vi "FileSend.vi"(8 "error in (no error)":errorcluster, 10 "(Empty=No Action)":path caption="File Name & Path", 11 "controller in":refnum<k24>) -> (0 "error out":errorcluster, 3 "controller out":refnum<k24>)   [LabVIEW 2010]
uses:
  c:/aerotech/controller/5.xx.xxx/ensemble/pc/labview/2010/bin/Aerotech.Ensemble.dll
  bin/Aerotech.Ensemble.dll
  c:/aerotech/controller/5.xx.xxx/ensemble/pc/labview/2010/bin/Aerotech.Ensemble.LabVIEW.dll
  bin/Aerotech.Ensemble.LabVIEW.dll
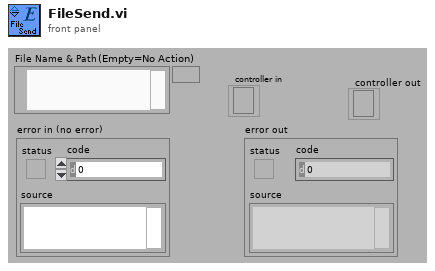
[diagram p1: front panel]
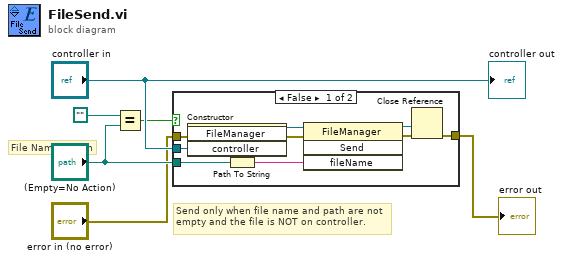
[diagram p0: block diagram]
diagram:
  # "File Name & Path"
  # "Send only when file name and path are not empty and the file is NOT on controller."
  n1 = Equal?(x=path "", y="(Empty=No Action)") -> (x = y?=w1:bool)
  n2 = case shown="False" w1 {
    tunnel: [w13 w16] -> w6
    tunnel: "(Empty=No Action)" -> [w12 _]
    tunnel: "error in (no error)" -> [w10 w16]
    tunnel: "controller in" -> [w9 _]
    frame False {
      n3 = constructor class="FileManager"(error in=w10, "controller"=w9) -> (reference out=w8:refnum<k24>, error out=w11:errorcluster)  [unwired: 2 in, 2 out]
      n4 = Path To String(path=w12) -> (string=w7:string)
      n5 = invoke class="FileManager" method="Send"(reference=w8, error in=w11, "fileName"=w7) -> (reference out=w14:refnum<k24>, error out=w15:errorcluster)  [unwired: 1 in, 2 out]
      n6 = Close Reference(reference=w14, error in (no error)=w15) -> (error out=w13:errorcluster)
    }
    frame True {
    }
  }
  "error out" <- w6
  "controller out" <- "controller in"
